vi "Kommunikation Stoerung.vi"(6 "Aktionen":T2, 8 "error in":errorcluster caption="Fehler (Eingang, kein Fehler)", 10 "ERROR":bool) -> (2 "Störung Messgerät":T1)   [LabVIEW 2020, in "Stoerungen.lvlib"]
uses:
  Stoerungen.lvlib
  Aktionen Kommunikation Stoerung.ctl
  Stoerungen Messgeraete.ctl
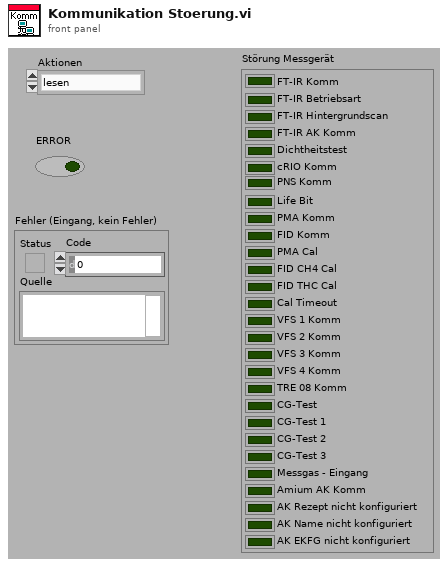
[diagram p1: front panel]
types:
  T1 = typedef "Stoerungen.lvlib/Stoerungen Messgeraete.ctl" = cluster{"FT-IR Komm":bool, "FT-IR Betriebsart":bool, "FT-IR Hintergrundscan":bool, "Dichtheitstest":bool, "cRIO Komm":bool, "PNS Komm":bool, "Life Bit":bool, "FT-IR AK Komm":bool, "PMA Komm":bool, "FID Komm":bool, "PMA Cal":bool, "FID CH4 Cal":bool, "FID THC Cal":bool, "Cal Timeout":bool, "VFS 1 Komm":bool, "VFS 2 Komm":bool, "VFS 3 Komm":bool, "VFS 4 Komm":bool, "TRE 08 Komm":bool, "CG-Test":bool, "CG-Test 1":bool, "CG-Test 2":bool, "CG-Test 3":bool, "Messgas - Eingang":bool, "Amium AK Komm":bool, "AK Rezept nicht konfiguriert ":bool, "AK Name nicht konfiguriert":bool, "AK EKFG nicht konfiguriert":bool}
  T2 = typedef "Stoerungen.lvlib/Aktionen Kommunikation Stoerung.ctl" = enum16{"lesen", "init", "FT-IR Komm", "FT-IR Betriebsart", "FT-IR Hintergrund", "cRIO Komm", "PNS Komm", "Dichtheitstest", "Life Bit", "FTIR Komm AK", "PMA Komm", "FID Komm", "PMA Cal", "FID Ch4 Cal", "FID THC Cal", "Cal Timeout", "VFS 1 Komm", "VFS 2 Komm", "VFS 3 Komm", "VFS 4 Komm", "TRE 08 Komm", "CG-Test vorzeitig", "CG-Test Span 1", "CG-Test Span 2", "CG-Test Span 3", "CG-Test Messgas", "CG-Test löschen", "Test", "Amium AK", "AK Recept konfig", "AK Name konfig", "AK EKFG konfig"}
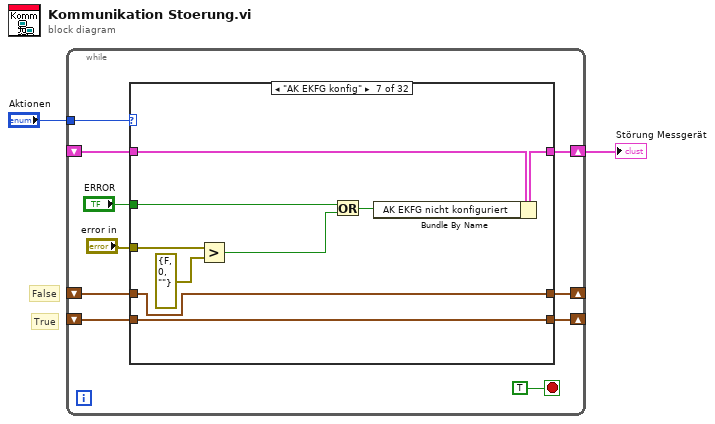
[diagram p0: block diagram]
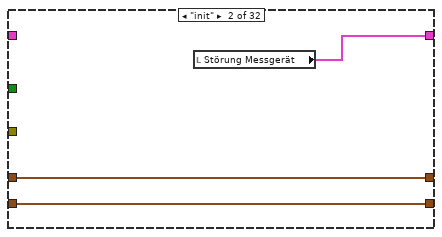
[diagram p3: hidden frame]
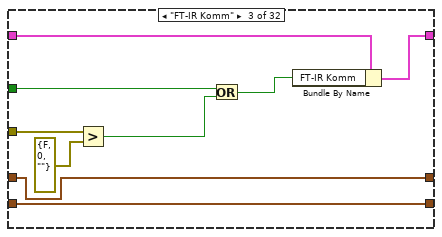
[diagram p4: hidden frame]
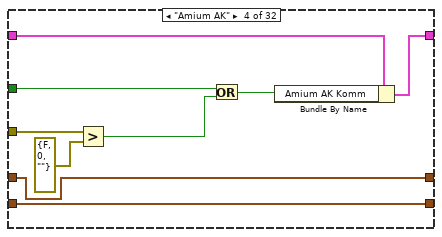
[diagram p5: hidden frame]
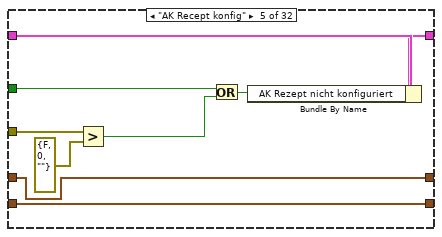
[diagram p6: hidden frame]
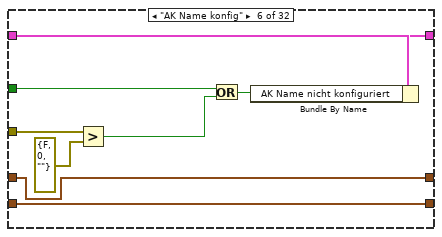
[diagram p7: hidden frame]
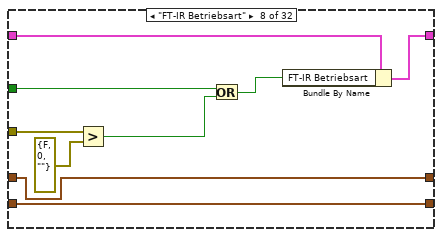
[diagram p8: hidden frame]
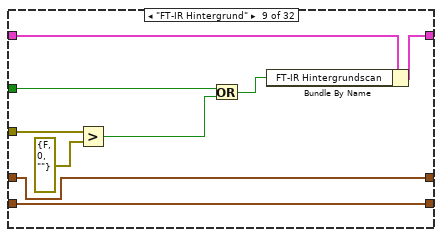
[diagram p9: hidden frame]
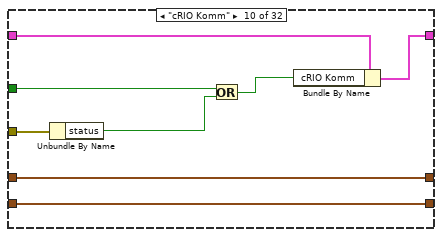
[diagram p10: hidden frame]
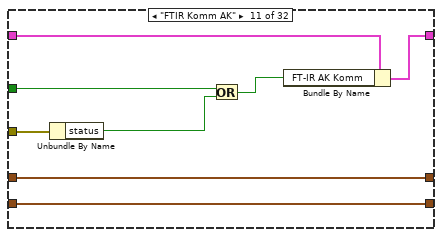
[diagram p11: hidden frame]
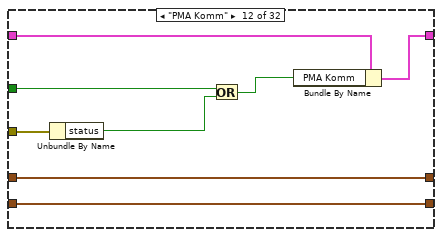
[diagram p12: hidden frame]
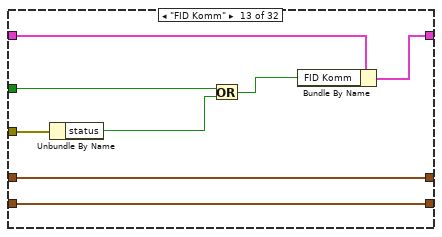
[diagram p13: hidden frame]
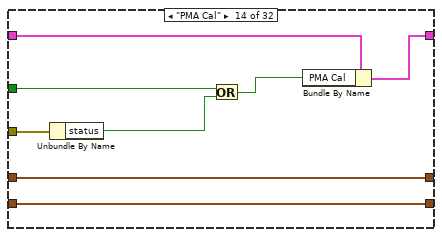
[diagram p14: hidden frame]
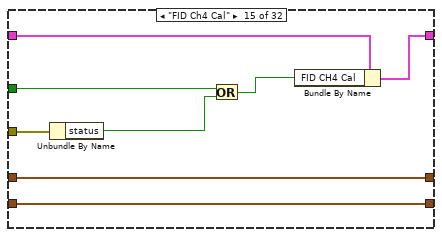
[diagram p15: hidden frame]
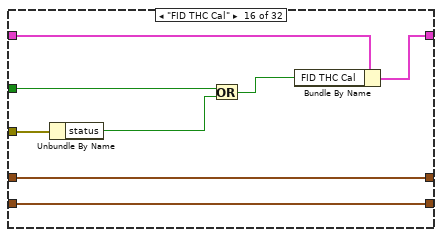
[diagram p16: hidden frame]
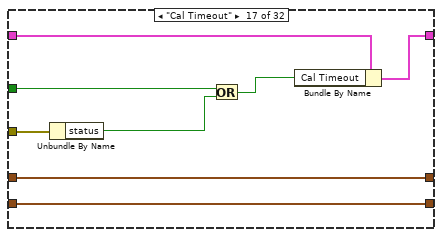
[diagram p17: hidden frame]
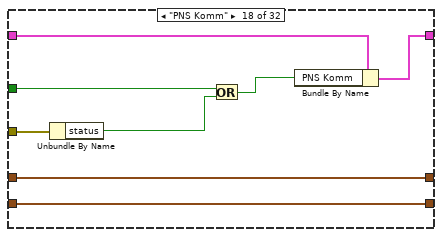
[diagram p18: hidden frame]
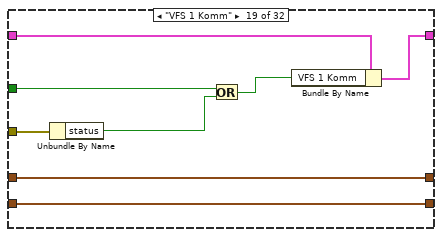
[diagram p19: hidden frame]
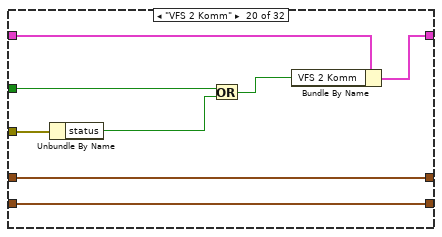
[diagram p20: hidden frame]
diagram:
  # "True"
  # "False"
  n1 = while {
    tunnel: "Aktionen" -> [w11]
    shift-right: [w8] -> w1
    shift-left: _ -> [w7]
    shift-right: [w6] -> _
    shift-left: _ -> [w3]
    shift-right: [w5] -> _
    shift-left: _ -> [w4]
    stop <- TRUE stop-if-true
    n2 = case shown="\"AK EKFG konfig\"" w11 {
      tunnel: "error in" -> [_ _ w26 w35 w44 w53 w62 w71 w80 w85 w93 w101 w109 w117 w125 w133 w141 w149 w157 w165 w173 w181 w189 w197 w205 w213 w221 w229 w237 w246 w253 w258]
      tunnel: "ERROR" -> [_ _ w25 w34 w43 w52 w61 w70 w79 w89 w97 w105 w113 w121 w129 w137 w145 w153 w161 w169 w177 w185 w193 w201 w209 w217 w225 w233 w241 w249 w257 w259]
      tunnel: [w15 w18 w22 w31 w40 w49 w58 w67 w76 w86 w94 w102 w110 w118 w126 w134 w142 w150 w158 w166 w174 w182 w190 w198 w206 w214 w222 w230 w238 w247 w254 w265] -> w8
      tunnel: w7 -> [w15 _ w24 w33 w42 w51 w60 w69 w78 w88 w96 w104 w112 w120 w128 w136 w144 w152 w160 w168 w176 w184 w192 w200 w208 w216 w224 w232 w240 w248 w256 w266]
      tunnel: [w14 w17 w20 w29 w38 w47 w56 w65 w74 w83 w91 w99 w107 w115 w123 w131 w139 w147 w155 w163 w171 w179 w187 w195 w203 w211 w219 w227 w235 w244 w251 w264] -> w6
      tunnel: [w13 w16 w19 w28 w37 w46 w55 w64 w73 w82 w90 w98 w106 w114 w122 w130 w138 w146 w154 w162 w170 w178 w186 w194 w202 w210 w218 w226 w234 w243 w250 w263] -> w5
      tunnel: w4 -> [w13 w16 w19 w28 w37 w46 w55 w64 w73 w82 w90 w98 w106 w114 w122 w130 w138 w146 w154 w162 w170 w178 w186 w194 w202 w210 w218 w226 w234 w243 w250 w262]
      tunnel: w3 -> [w14 w17 w20 w29 w38 w47 w56 w65 w74 w83 w91 w99 w107 w115 w123 w131 w139 w147 w155 w163 w171 w179 w187 w195 w203 w211 w219 w227 w235 w244 w251 w261]
      frame "lesen", Default {
      }
      frame "init" {
        n3 = local read "Störung Messgerät"() -> (w18:T1)
      }
      frame "FT-IR Komm" {
        n4 = Greater?(x=w26, y=errorcluster {"status"=FALSE, "code"=0, "source"=""}) -> (0:w21:bool)
        n5 = Or(x=w25, y=w21) -> (x .or. y?=w23:bool)
        n6 = Bundle By Name(cluster=w24, "FT-IR Komm"=w23) -> (w22:T1)
      }
      frame "Amium AK" {
        n7 = Greater?(x=w35, y=errorcluster {"status"=FALSE, "code"=0, "source"=""}) -> (0:w30:bool)
        n8 = Or(x=w34, y=w30) -> (x .or. y?=w32:bool)
        n9 = Bundle By Name(cluster=w33, "Amium AK Komm"=w32) -> (w31:T1)
      }
      frame "AK Recept konfig" {
        n10 = Greater?(x=w44, y=errorcluster {"status"=FALSE, "code"=0, "source"=""}) -> (0:w39:bool)
        n11 = Or(x=w43, y=w39) -> (x .or. y?=w41:bool)
        n12 = Bundle By Name(cluster=w42, "AK Rezept nicht konfiguriert"=w41) -> (w40:T1)
      }
      frame "AK Name konfig" {
        n13 = Greater?(x=w53, y=errorcluster {"status"=FALSE, "code"=0, "source"=""}) -> (0:w48:bool)
        n14 = Or(x=w52, y=w48) -> (x .or. y?=w50:bool)
        n15 = Bundle By Name(cluster=w51, "AK Name nicht konfiguriert"=w50) -> (w49:T1)
      }
      frame "AK EKFG konfig" {
        n16 = Greater?(x=w62, y=errorcluster {"status"=FALSE, "code"=0, "source"=""}) -> (0:w57:bool)
        n17 = Or(x=w61, y=w57) -> (x .or. y?=w59:bool)
        n18 = Bundle By Name(cluster=w60, "AK EKFG nicht konfiguriert"=w59) -> (w58:T1)
      }
      frame "FT-IR Betriebsart" {
        n19 = Greater?(x=w71, y=errorcluster {"status"=FALSE, "code"=0, "source"=""}) -> (0:w66:bool)
        n20 = Or(x=w70, y=w66) -> (x .or. y?=w68:bool)
        n21 = Bundle By Name(cluster=w69, "FT-IR Betriebsart"=w68) -> (w67:T1)
      }
      frame "FT-IR Hintergrund" {
        n22 = Greater?(x=w80, y=errorcluster {"status"=FALSE, "code"=0, "source"=""}) -> (0:w75:bool)
        n23 = Or(x=w79, y=w75) -> (x .or. y?=w77:bool)
        n24 = Bundle By Name(cluster=w78, "FT-IR Hintergrundscan"=w77) -> (w76:T1)
      }
      frame "cRIO Komm" {
        n25 = Unbundle By Name(w85) -> ("status"=w84:bool)
        n26 = Or(x=w89, y=w84) -> (x .or. y?=w87:bool)
        n27 = Bundle By Name(cluster=w88, "cRIO Komm"=w87) -> (w86:T1)
      }
      frame "FTIR Komm AK" {
        n28 = Unbundle By Name(w93) -> ("status"=w92:bool)
        n29 = Or(x=w97, y=w92) -> (x .or. y?=w95:bool)
        n30 = Bundle By Name(cluster=w96, "FT-IR AK Komm"=w95) -> (w94:T1)
      }
      frame "PMA Komm" {
        n31 = Unbundle By Name(w101) -> ("status"=w100:bool)
        n32 = Or(x=w105, y=w100) -> (x .or. y?=w103:bool)
        n33 = Bundle By Name(cluster=w104, "PMA Komm"=w103) -> (w102:T1)
      }
      frame "FID Komm" {
        n34 = Unbundle By Name(w109) -> ("status"=w108:bool)
        n35 = Or(x=w113, y=w108) -> (x .or. y?=w111:bool)
        n36 = Bundle By Name(cluster=w112, "FID Komm"=w111) -> (w110:T1)
      }
      frame "PMA Cal" {
        n37 = Unbundle By Name(w117) -> ("status"=w116:bool)
        n38 = Or(x=w121, y=w116) -> (x .or. y?=w119:bool)
        n39 = Bundle By Name(cluster=w120, "PMA Cal"=w119) -> (w118:T1)
      }
      frame "FID Ch4 Cal" {
        n40 = Unbundle By Name(w125) -> ("status"=w124:bool)
        n41 = Or(x=w129, y=w124) -> (x .or. y?=w127:bool)
        n42 = Bundle By Name(cluster=w128, "FID CH4 Cal"=w127) -> (w126:T1)
      }
      frame "FID THC Cal" {
        n43 = Unbundle By Name(w133) -> ("status"=w132:bool)
        n44 = Or(x=w137, y=w132) -> (x .or. y?=w135:bool)
        n45 = Bundle By Name(cluster=w136, "FID THC Cal"=w135) -> (w134:T1)
      }
      frame "Cal Timeout" {
        n46 = Unbundle By Name(w141) -> ("status"=w140:bool)
        n47 = Or(x=w145, y=w140) -> (x .or. y?=w143:bool)
        n48 = Bundle By Name(cluster=w144, "Cal Timeout"=w143) -> (w142:T1)
      }
      frame "PNS Komm" {
        n49 = Unbundle By Name(w149) -> ("status"=w148:bool)
        n50 = Or(x=w153, y=w148) -> (x .or. y?=w151:bool)
        n51 = Bundle By Name(cluster=w152, "PNS Komm"=w151) -> (w150:T1)
      }
      frame "VFS 1 Komm" {
        n52 = Unbundle By Name(w157) -> ("status"=w156:bool)
        n53 = Or(x=w161, y=w156) -> (x .or. y?=w159:bool)
        n54 = Bundle By Name(cluster=w160, "VFS 1 Komm"=w159) -> (w158:T1)
      }
      frame "VFS 2 Komm" {
        n55 = Unbundle By Name(w165) -> ("status"=w164:bool)
        n56 = Or(x=w169, y=w164) -> (x .or. y?=w167:bool)
        n57 = Bundle By Name(cluster=w168, "VFS 2 Komm"=w167) -> (w166:T1)
      }
      frame "VFS 3 Komm" {
        n58 = Unbundle By Name(w173) -> ("status"=w172:bool)
        n59 = Or(x=w177, y=w172) -> (x .or. y?=w175:bool)
        n60 = Bundle By Name(cluster=w176, "VFS 3 Komm"=w175) -> (w174:T1)
      }
      frame "VFS 4 Komm" {
        n61 = Unbundle By Name(w181) -> ("status"=w180:bool)
        n62 = Or(x=w185, y=w180) -> (x .or. y?=w183:bool)
        n63 = Bundle By Name(cluster=w184, "VFS 4 Komm"=w183) -> (w182:T1)
      }
      frame "TRE 08 Komm" {
        n64 = Unbundle By Name(w189) -> ("status"=w188:bool)
        n65 = Or(x=w193, y=w188) -> (x .or. y?=w191:bool)
        n66 = Bundle By Name(cluster=w192, "TRE 08 Komm"=w191) -> (w190:T1)
      }
      frame "CG-Test vorzeitig" {
        n67 = Unbundle By Name(w197) -> ("status"=w196:bool)
        n68 = Or(x=w201, y=w196) -> (x .or. y?=w199:bool)
        n69 = Bundle By Name(cluster=w200, "CG-Test"=w199) -> (w198:T1)
      }
      frame "Test" {
        n70 = Unbundle By Name(w205) -> ("status"=w204:bool)
        n71 = Or(x=w209, y=w204) -> (x .or. y?=w207:bool)
        n72 = Bundle By Name(cluster=w208, "TRE 08 Komm"=w207) -> (w206:T1)
      }
      frame "CG-Test Span 1" {
        n73 = Unbundle By Name(w213) -> ("status"=w212:bool)
        n74 = Or(x=w217, y=w212) -> (x .or. y?=w215:bool)
        n75 = Bundle By Name(cluster=w216, "CG-Test 1"=w215) -> (w214:T1)
      }
      frame "CG-Test Span 2" {
        n76 = Unbundle By Name(w221) -> ("status"=w220:bool)
        n77 = Or(x=w225, y=w220) -> (x .or. y?=w223:bool)
        n78 = Bundle By Name(cluster=w224, "CG-Test 2"=w223) -> (w222:T1)
      }
      frame "CG-Test Span 3" {
        n79 = Unbundle By Name(w229) -> ("status"=w228:bool)
        n80 = Or(x=w233, y=w228) -> (x .or. y?=w231:bool)
        n81 = Bundle By Name(cluster=w232, "CG-Test 3"=w231) -> (w230:T1)
      }
      frame "CG-Test Messgas" {
        n82 = Unbundle By Name(w237) -> ("status"=w236:bool)
        n83 = Or(x=w241, y=w236) -> (x .or. y?=w239:bool)
        n84 = Bundle By Name(cluster=w240, "Messgas - Eingang"=w239) -> (w238:T1)
      }
      frame "CG-Test löschen" {
        n85 = Unbundle By Name(w246) -> ("status"=w245:bool)
        n86 = Or(x=w249, y=w245) -> (x .or. y?=w242:bool)
        n87 = Bundle By Name(cluster=w248, "CG-Test"=w242, "CG-Test 1"=w242, "CG-Test 2"=w242, "CG-Test 3"=w242, "Messgas - Eingang"=w242) -> (w247:T1)
      }
      frame "Dichtheitstest" {
        n88 = Unbundle By Name(w253) -> ("status"=w252:bool)
        n89 = Or(x=w257, y=w252) -> (x .or. y?=w255:bool)
        n90 = Bundle By Name(cluster=w256, "Dichtheitstest"=w255) -> (w254:T1)
      }
      frame "Life Bit" {
        n91 = call <vilib>:"Clear Errors.vi"("error in (no error)"=w258) -> ()  [unwired: 5 in, 2 out]
        n92 = case shown="False" w259 {
          tunnel: w262 -> [_ w275]
          tunnel: w261 -> [w268 _]
          tunnel: [w268 w276] -> w264
          tunnel: [w269 w275] -> w263
          tunnel: [w267 w272] -> w260
          frame False {
            n93 = Get Date/Time In Seconds() -> (seconds since 1Jan1904=w269:timestamp)
            n94 = Subtract(x=w269, y=w268) -> (x-y=w271:dbl)
            n95 = Greater?(x=w271, y=20.0) -> (0:w267:bool)
          }
          frame True {
            n96 = Get Date/Time In Seconds() -> (seconds since 1Jan1904=w276:timestamp)
            n97 = Subtract(x=w276, y=w275) -> (x-y=w274:dbl)
            n98 = Greater?(x=w274, y=20.0) -> (0:w272:bool)
          }
        }
        n99 = Bundle By Name(cluster=w266, "Life Bit"=w260) -> (w265:T1)
      }
    }
  }
  "Störung Messgerät" <- w1
